vi "IsProxy.vi"(8 "error in (no error)":errorcluster, 11 "Subject in":refnum<class "Subject.lvclass">) -> (0 "error out":errorcluster, 2 "isProxy?":bool, 3 "Subject out":refnum<class "Subject.lvclass">)   [LabVIEW 2014, in "forcible Proxy.lvlib" / "Subject.lvclass"]
uses:
  Subject.lvclass
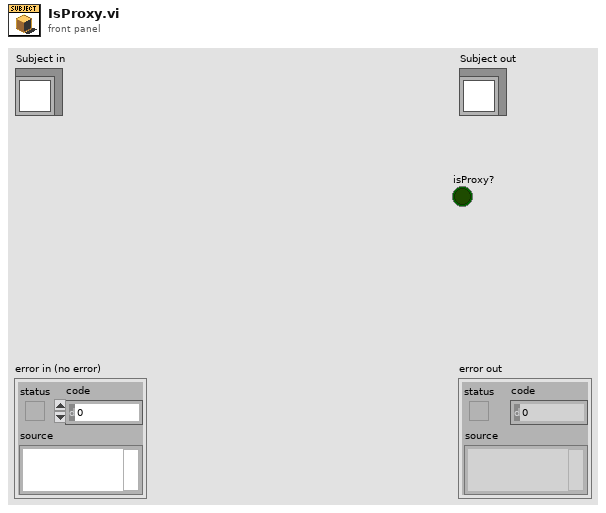
[diagram p1: front panel]
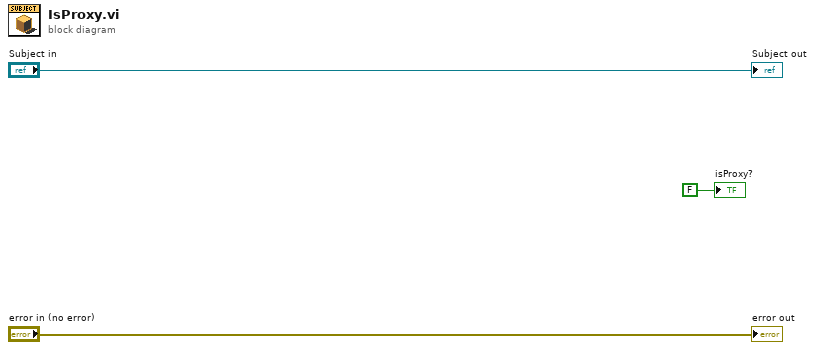
[diagram p0: block diagram]
diagram:
  "error out" <- "error in (no error)"
  "Subject out" <- "Subject in"
  "isProxy?" <- FALSE
